vi "setControlSensor.vi"(8 "error in (no error)":errorcluster, 10 "ControlSensor in":T2, 11 "CoolerControler in":refnum<class "CoolerControler.lvclass">) -> (0 "error out":errorcluster, 2 "ControlSensor out":T2, 3 "CoolerControler out":refnum<class "CoolerControler.lvclass">)   [LabVIEW 2016, in "CoolerControler.lvclass"]
uses:
  CoolerControler.lvclass
  typedefs/ControlSensor.ctl
  typedefs/CoolerId.ctl
  SerialCommand/CoolerSerialCommand.lvclass
  typedefs/dataUnit.ctl
  typedefs/CoolerCommands.ctl
panel:
  in  "id":T1=1
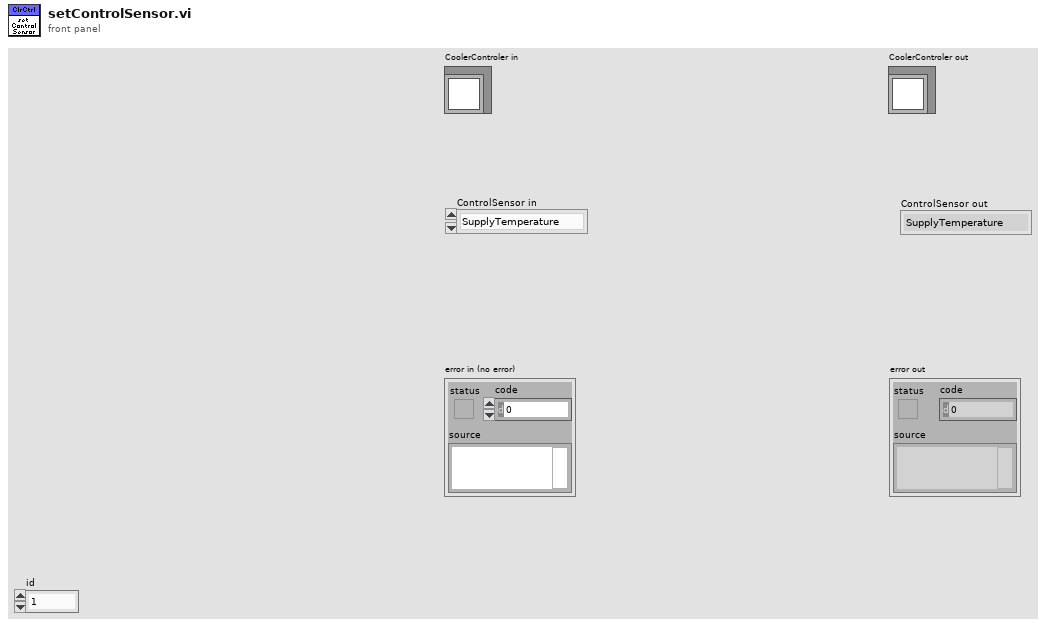
[diagram p1: front panel]
types:
  T1 = typedef "CoolerId.ctl" = u16
  T2 = typedef "ControlSensor.ctl" = enum16{"SupplyTemperature", "ReturnTemperature", "ExtRTD", "ExternalTermistor"}
  T3 = typedef "CoolerCommands.ctl" = enum16{"None", "SetExternSensorStatus", "SetChillerStatus", "SetControlSensor", "SetControlTemperature", "SetHighSupplyTempWarning", "SetLowSupplyTemperatureWarning", "SetHighAmbientTemperatureWarning", "SetLowAmbienTemperatureWarning", "SetLowProcessFlowWarning", "SetHighSupplyTemperatureAlarm", "SetLowSupplyTemperatureAlarm", "SetHighAmbientTemperatureAlarm", "SetLowAmbientTemperatureAlarm", "SetLowProcessFlowAlarm"}
  T4 = typedef "dataUnit.ctl" = enum16{"temperature", "flow", "current", "PID", "fanSpeed", "time", "PWM", "TEDriveLevel", "Number"}
  T5 = typedef "response.ctl" = cluster{"deviceId":string, "commandNumber":string, "errorActive":bool, "commandName":string, "responseData":string, "checkSum":string}
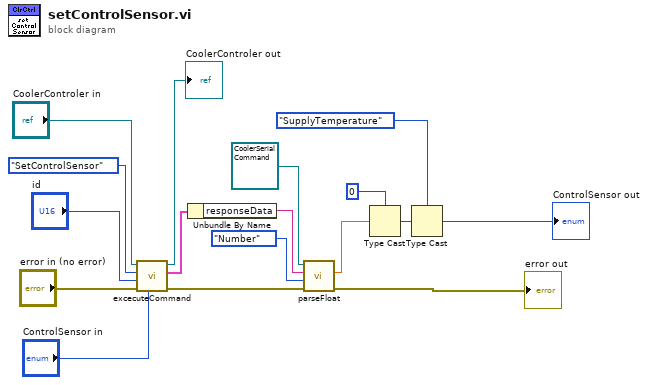
[diagram p0: block diagram]
diagram:
  n1 = call "excecuteCommand.vi"("inputValue"="ControlSensor in", "error in (no error)"="error in (no error)", "id"="id", "CoolerCommand"=CoolerCommands."SetControlSensor", "CoolerControler in"="CoolerControler in") -> ("error out"=w16:errorcluster, "response out"=w15:T5, "CoolerControler out"=→"CoolerControler out":refnum<class "CoolerControler.lvclass">)  [unwired: 4 in]
  n2 = Unbundle By Name(w15) -> ("responseData"=w13:string)
  n3 = call "parseFloat.vi"("error in (no error)"=w16, "unit"=dataUnit."Number", "commandData"=w13, "CoolerSerialCommand in"=refnum<class "CoolerSerialCommand.lvclass"> refnum) -> ("error out"=→"error out":errorcluster, "value"=w3:sgl)  [unwired: 4 in, 2 out]
  n4 = Type Cast(type=u16 0, x=w3) -> (*(type *) &x=w5:u16)
  n5 = Type Cast(type=ControlSensor."SupplyTemperature" ("ControlSensor out"), x=w5) -> (*(type *) &x=→"ControlSensor out":T2)
